vi "ConsumerProducer.vi"() -> ()   [LabVIEW 2011]
panel:
  out "error out 1":errorcluster
  out "error out 2":errorcluster
  out "error out 3":errorcluster
  out "error out":errorcluster caption="Fehler (Ausgang)"
  out "Loop3 Verbliebene Elemente":dbl[](array[numeric])
  out "Loop2 Verbliebene Elemente":dbl[](array[numeric])
  out "Loop1 Verbliebene Elemente":dbl[](array[numeric])
  out "Loop3 elements":i32
  out "Loop2 elements":i32
  out "Loop1 elements":i32
  in  "Consumer timer":u32=1000
  out "Consumer data":dbl
  out "Loop3 data":dbl
  out "Loop2 data":dbl
  out "Loop1 data":dbl
  in  "Loop3 timer":u32=1000
  in  "Loop2 timer":u32=1000
  in  "Loop1 timer":u32=1000
  in  "Stopp":bool
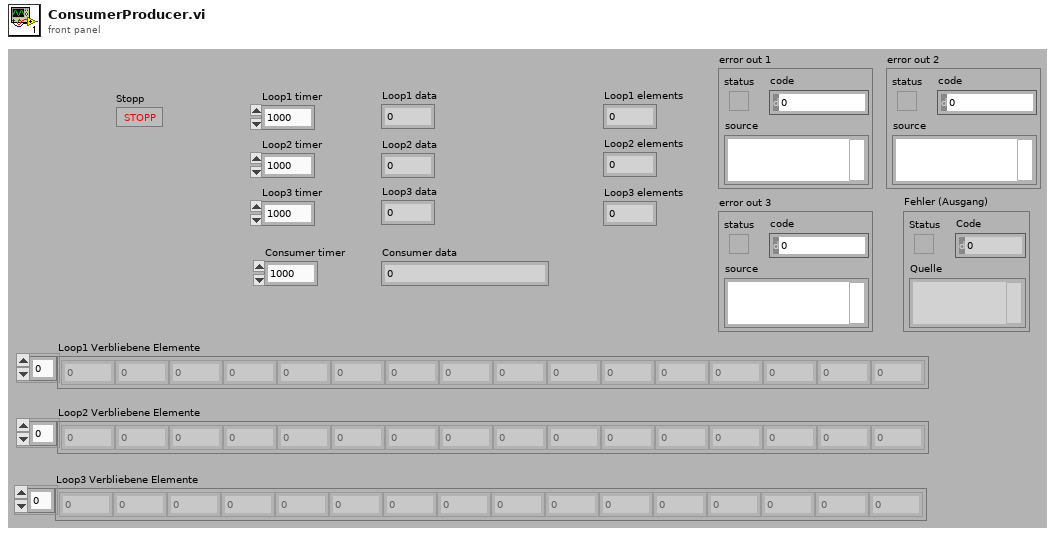
[diagram p1: front panel]
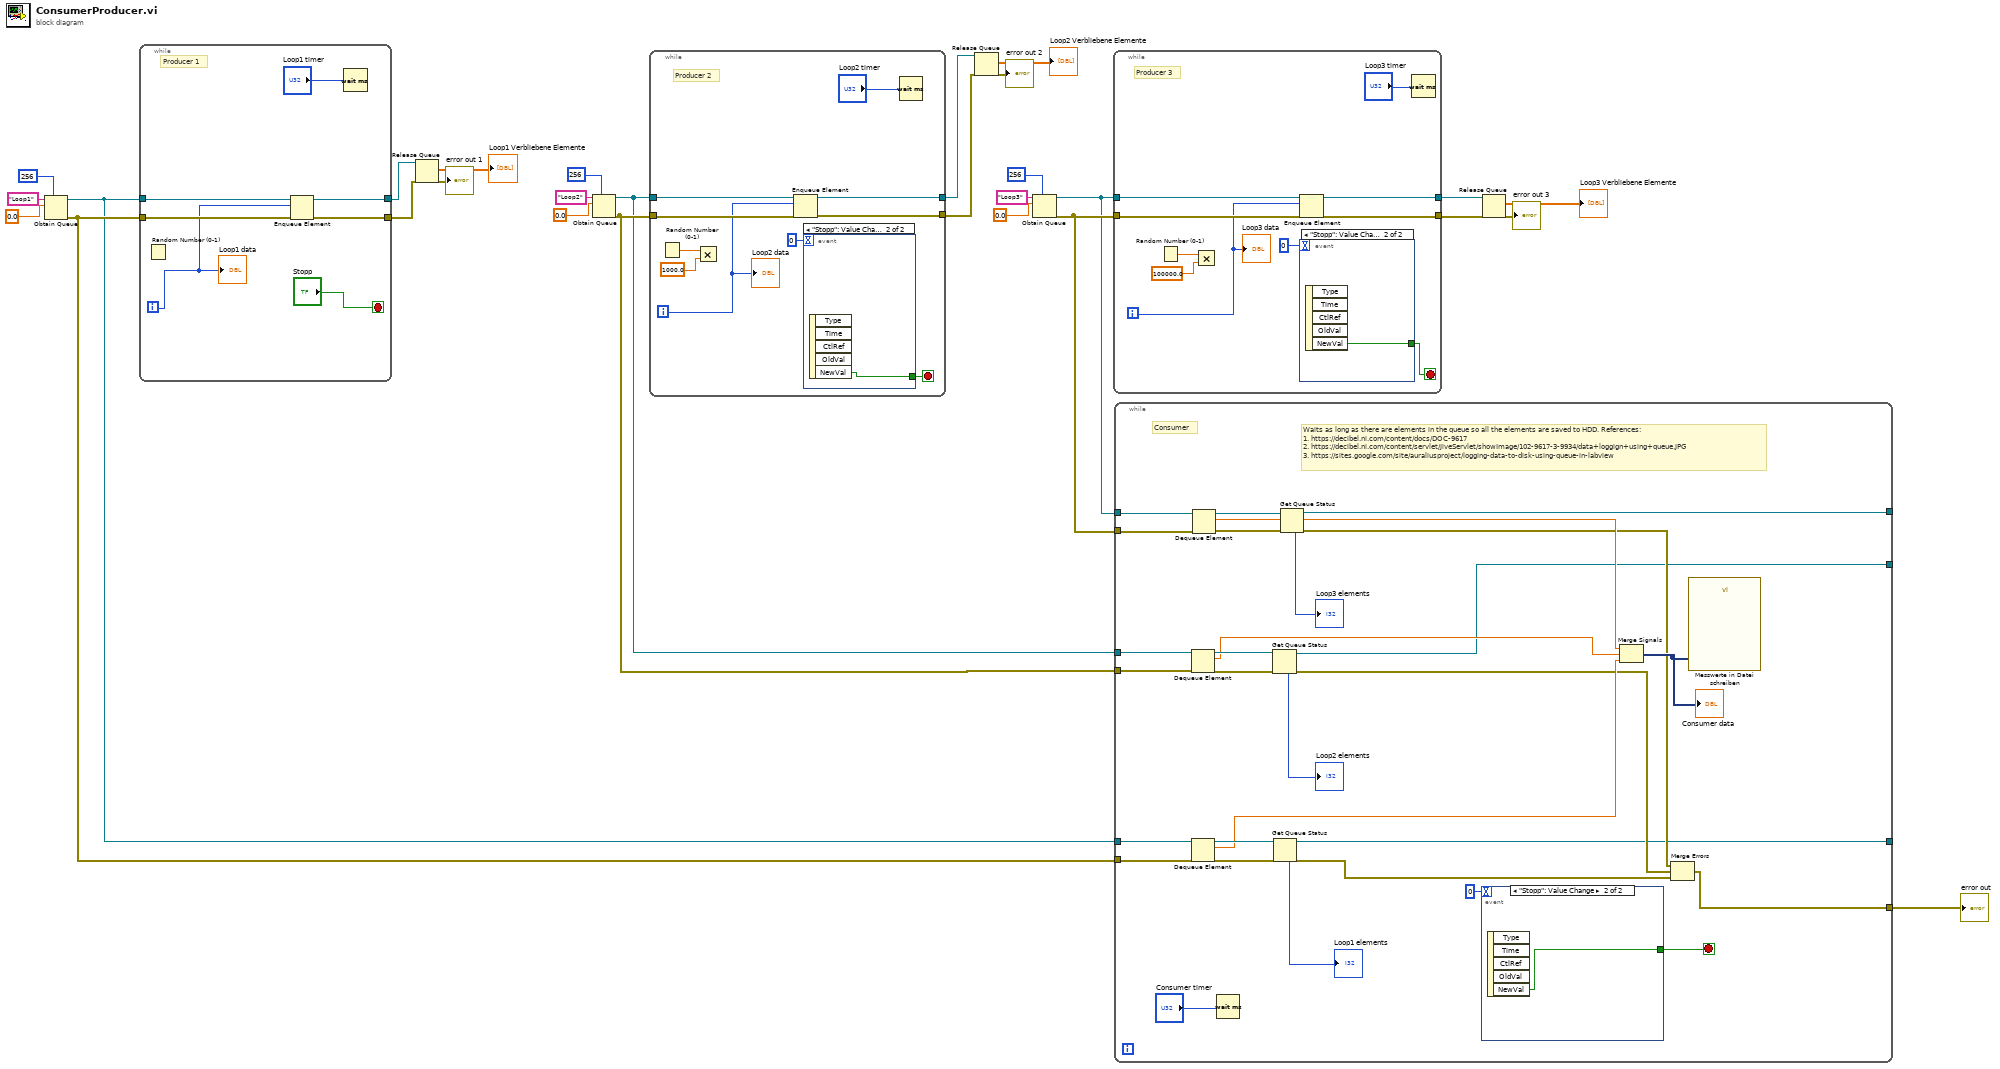
[diagram p0: block diagram]
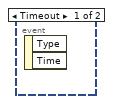
[diagram p2: hidden frame]
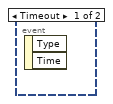
[diagram p3: hidden frame]
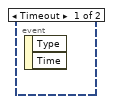
[diagram p4: hidden frame]
diagram:
  n1 = Obtain Queue(max queue size (-1, unlimited)=256, name (unnamed)="Loop1" ("Name (unbenannt)"), element data type=0.0 ("Wert (0 bis 1)")) -> (queue out=w17:refnum<queue>, error out=w22:errorcluster)  [unwired: 2 in, 1 out]
  n2 = while {
    tunnel: w17 -> [w35]
    tunnel: [w34] -> w5
    tunnel: w22 -> [w33]
    tunnel: [w31] -> w4
    i -> [w30]
    stop <- "Stopp" stop-if-true
    # "Producer 1"
    n3 = Random Number (0-1)() -> ()  [unwired: 1 out]
    n4 = Enqueue Element(queue=w35, element=w30, error in (no error)=w33) -> (queue out=w34:refnum<queue>, error out=w31:errorcluster)  [unwired: 2 out]
    n5 = Wait (ms)(milliseconds to wait="Loop1 timer") -> ()  [unwired: 1 out]
    "Loop1 data" <- w30
  }
  n6 = Release Queue(queue=w5, error in (no error)=w4) -> (remaining elements=→"Loop1 Verbliebene Elemente":dbl[], error out=→"error out 1":errorcluster)  [unwired: 2 out]
  n7 = Obtain Queue(max queue size (-1, unlimited)=256, name (unnamed)="Loop2" ("Name (unbenannt)"), element data type=0.0 ("Wert (0 bis 1)")) -> (queue out=w15:refnum<queue>, error out=w21:errorcluster)  [unwired: 2 in, 1 out]
  n8 = while {
    tunnel: w15 -> [w45]
    tunnel: w21 -> [w44]
    tunnel: [w43] -> w8
    tunnel: [w39] -> w7
    i -> [w38]
    stop <- w37 stop-if-true
    # "Producer 2"
    n9 = Random Number (0-1)() -> (number: 0 to 1=w42:dbl)
    n10 = Multiply(x=w42, y=1000.0) -> ()  [unwired: 1 out]
    n11 = Enqueue Element(queue=w45, element=w38, error in (no error)=w44) -> (queue out=w43:refnum<queue>, error out=w39:errorcluster)  [unwired: 2 out]
    n12 = event shown="[1] \"Stopp\": Value Change" {
      selector: _ -> [_ _]
      dyn-events: _ -> [_ _]
      timeout: 0 -> [_ _]
      tunnel: [_ w46] -> w37
      event Timeout {
        n13 = event-data() -> ()  [unwired: 1 in, 2 out]
      }
      event "Stopp": Value Change {
        n14 = event-data() -> ("NewVal"=w46:bool)  [unwired: 1 in, 4 out]
      }
    }
    n15 = Wait (ms)(milliseconds to wait="Loop2 timer") -> ()  [unwired: 1 out]
    "Loop2 data" <- w38
  }
  n16 = Release Queue(queue=w8, error in (no error)=w7) -> (remaining elements=→"Loop2 Verbliebene Elemente":dbl[], error out=→"error out 2":errorcluster)  [unwired: 2 out]
  n17 = Obtain Queue(max queue size (-1, unlimited)=256, name (unnamed)="Loop3" ("Name (unbenannt)"), element data type=0.0 ("Wert (0 bis 1)")) -> (queue out=w16:refnum<queue>, error out=w20:errorcluster)  [unwired: 2 in, 1 out]
  n18 = while {
    tunnel: w16 -> [w56]
    tunnel: [w55] -> w10
    tunnel: w20 -> [w54]
    tunnel: [w49] -> w9
    i -> [w50]
    stop <- w48 stop-if-true
    # "Producer 3"
    n19 = Random Number (0-1)() -> (number: 0 to 1=w53:dbl)
    n20 = Multiply(x=w53, y=100000.0) -> ()  [unwired: 1 out]
    n21 = Enqueue Element(queue=w56, element=w50, error in (no error)=w54) -> (queue out=w55:refnum<queue>, error out=w49:errorcluster)  [unwired: 2 out]
    n22 = event shown="[1] \"Stopp\": Value Change" {
      selector: _ -> [_ _]
      dyn-events: _ -> [_ _]
      timeout: 0 -> [_ _]
      tunnel: [_ w57] -> w48
      event Timeout {
        n23 = event-data() -> ()  [unwired: 1 in, 2 out]
      }
      event "Stopp": Value Change {
        n24 = event-data() -> ("NewVal"=w57:bool)  [unwired: 1 in, 4 out]
      }
    }
    n25 = Wait (ms)(milliseconds to wait="Loop3 timer") -> ()  [unwired: 1 out]
    "Loop3 data" <- w50
  }
  n26 = while {
    tunnel: w17 -> [w81]
    tunnel: w15 -> [w86]
    tunnel: w16 -> [w85]
    tunnel: w22 -> [w80]
    tunnel: w21 -> [w79]
    tunnel: w20 -> [w78]
    tunnel: [w63] -> w14
    tunnel: [w62] -> _
    tunnel: [w61] -> _
    tunnel: [w60] -> _
    stop <- w59 stop-if-true
    # "Waits as long as there are elements in the queue so all the elements are saved to HDD. References:\n1. https://decibel.ni.com/content/docs/DOC-9617\n2. https://decibel.ni.com/content/servlet/JiveServlet/showImage/102-9617-3-9934/data+loggign+using+queue.JPG\n3. https://sites.google.com/site/auraliusproject/logging-data-to-disk-using-queue-in-labview"
    # "Consumer"
    n27 = Dequeue Element(queue=w86, error in (no error)=w79) -> (queue out=w72:refnum<queue>, element=w70:dbl, error out=w71:errorcluster)  [unwired: 2 out]
    n28 = Dequeue Element(queue=w81, error in (no error)=w80) -> (queue out=w77:refnum<queue>, element=w73:dbl, error out=w76:errorcluster)  [unwired: 2 out]
    n29 = Dequeue Element(queue=w85, error in (no error)=w78) -> (queue out=w69:refnum<queue>, element=w84:dbl, error out=w68:errorcluster)  [unwired: 2 out]
    n30 = Wait (ms)(milliseconds to wait="Consumer timer") -> ()  [unwired: 1 out]
    n31 = Get Queue Status(queue=w72, error in (no error)=w71) -> (queue out=w61:refnum<queue>, error out=w67:errorcluster, # elements in queue=→"Loop2 elements":i32)  [unwired: 6 out]
    n32 = Get Queue Status(queue=w77, error in (no error)=w76) -> (queue out=w62:refnum<queue>, error out=w75:errorcluster, # elements in queue=→"Loop1 elements":i32)  [unwired: 6 out]
    n33 = Get Queue Status(queue=w69, error in (no error)=w68) -> (queue out=w60:refnum<queue>, error out=w64:errorcluster, # elements in queue=→"Loop3 elements":i32)  [unwired: 6 out]
    n34 = event shown="[1] \"Stopp\": Value Change" {
      selector: _ -> [_ _]
      dyn-events: _ -> [_ _]
      timeout: 0 -> [_ _]
      tunnel: [_ w87] -> w59
      event Timeout {
        n35 = event-data() -> ()  [unwired: 1 in, 2 out]
      }
      event "Stopp": Value Change {
        n36 = event-data() -> ("NewVal"=w87:bool)  [unwired: 1 in, 4 out]
      }
    }
    n37 = Merge Signals(w84, w70, w73) -> (w83:dynamicdata)
    "Consumer data" <- w83
    n38 = Merge Errors(w64, w67, w75) -> (w63:errorcluster)
    n39 = call "Messwerte in Datei schreiben"("Signals"=w83) -> ()  [unwired: 6 in, 13 out]
  }
  "error out" <- w14
  n40 = Release Queue(queue=w10, error in (no error)=w9) -> (remaining elements=→"Loop3 Verbliebene Elemente":dbl[], error out=→"error out 3":errorcluster)  [unwired: 2 out]
